vi "Read Laser properties.vi"(8 "error in (no error)":errorcluster, 11 "HC-ScanParser in":refnum<class "HC-ScanParser.lvclass">) -> (0 "error out":errorcluster, 2 "Laser properties":T1={"MaximumLaserPower"=500.0, "Power curve"={"Watt"=[0.0, 500.0], "Bits"=[0, 255]}, "Rise time"=10, "Fall time"=10}, 3 "HC-ScanParser out":refnum<class "HC-ScanParser.lvclass">)   [LabVIEW 2013, in "HardwareCharacterization.lvlib" / "HC-ScanParser.lvclass"]
uses:
  HC-ScanParser.lvclass
  Laser-properties.ctl
  HC-ScanParser.lvclass/HC-ScanParser.ctl
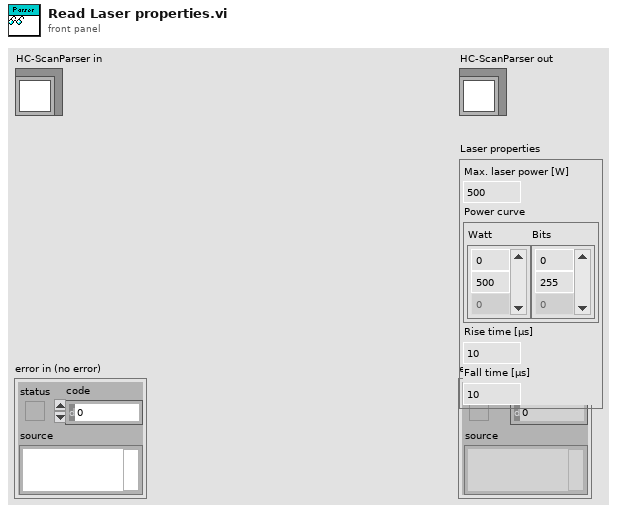
[diagram p1: front panel]
types:
  T1 = typedef "HardwareCharacterization.lvlib/HC-ScanParser.lvclass/Laser-properties.ctl" = cluster{"MaximumLaserPower":dbl, "Power curve":cluster{"Watt":dbl[], "Bits":u8[]}, "Rise time":i64, "Fall time":i64}
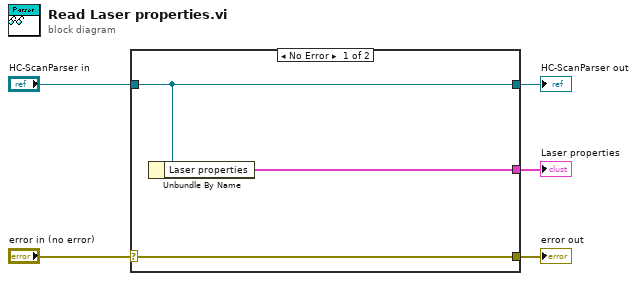
[diagram p0: block diagram]
diagram:
  n1 = case shown="No Error" "error in (no error)" {
    selector: "error in (no error)" -> [w8 w9]
    tunnel: [w8 w9] -> w4
    tunnel: [w7 w10] -> w2
    tunnel: "HC-ScanParser in" -> [w7 w10]
    tunnel: [w6 _] -> w1
    frame No Error {
      n2 = Unbundle By Name(w7) -> ("Laser properties"=w6:T1)
    }
    frame Error {
    }
  }
  "error out" <- w4
  "HC-ScanParser out" <- w2
  "Laser properties" <- w1
